vi "Update PrependMinionID.vi"(8 "Error In":errorcluster, 10 "PrependMinionID":bool, 11 "Data Value Reference in":refnum<data-value>) -> (0 "error out":errorcluster)   [LabVIEW 2015, in "SystemLink editor node.lvclass"]
doc: "Update module configuration class within Node Ref to new <b>PrependMinionID</b> value"
uses:
  SystemLink editor node.lvclass
  <vilib>/NI/DCAF/Tag Editor Core/Configuration Editor/Classes/Module editor node/module editor node.lvclass
  SystemLink editor node.lvclass/SystemLink editor node.ctl
  module/configuration/SystemLink configuration.lvclass/SystemLink configuration.ctl
  module/configuration/Write Prepend Minion ID.vi
  module/configuration/SystemLink configuration.lvclass
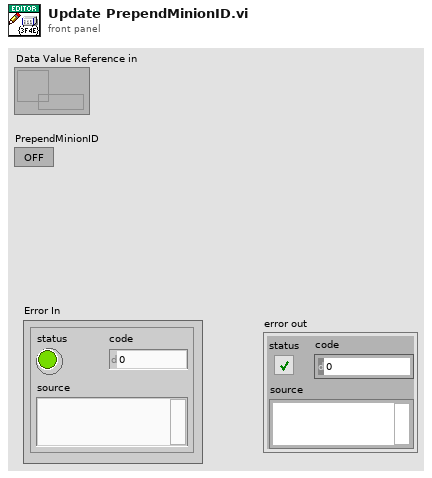
[diagram p1: front panel]
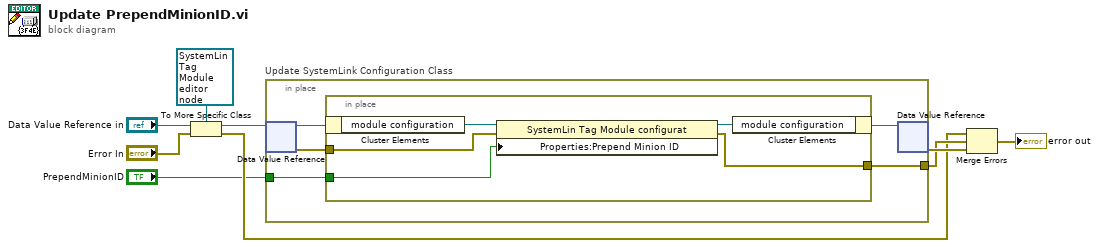
[diagram p0: block diagram]
diagram:
  n1 = To More Specific Class(target class=refnum<data-value> refnum ("Data Value Reference in"), reference="Data Value Reference in", error in="Error In") -> (specific class reference=w9:refnum<data-value>, error out=w5:errorcluster)
  n2 = in-place "Update SystemLink Configuration Class" {
    in-place-border: [w11] -> w6
    in-place-border: "PrependMinionID" -> [w10]
    n3 = in-place-dvr #1(w9) -> (w14:refnum<class "SystemLink editor node.lvclass">, w12:errorcluster)
    n4 = in-place {
      in-place-border: w12 -> [w17]
      in-place-border: [w16] -> w11
      in-place-border: w10 -> [w15]
      n5 = in-place-cluster #2(w14) -> ("module configuration"=w19:refnum<class "SystemLink configuration.lvclass">)
      n6 = property class="SystemLin Tag Module configurat"(reference=w19, error in=w17, "Properties:Prepend Minion ID"=w15) -> (reference out=w18:refnum<class "SystemLink configuration.lvclass">, error out=w16:errorcluster)
      n7 = in-place-cluster #2("module configuration"=w18) -> (w13:refnum<class "SystemLink editor node.lvclass">)
    }
    n8 = in-place-dvr #1(w13) -> (w7:errorcluster)  [unwired: 1 out]
  }
  n9 = Merge Errors(w5, w6, w7) -> (→"error out":errorcluster)
